vi "autolock.vi"   [LabVIEW 2012]
uses:
  Robot Global Data.vi
  <vilib>/Rock Robotics/WPI/RobotDrive/WPI_RobotDriveGetSetRefNum.vi
types:
  T1 = cluster{"Position":cluster{"X":i32, "Y":i32}, "Distance (ft)":i32, "Center":bool, "Top":bool, "Mid":bool}
  T2 = cluster{"Center Position":cluster{"X":dbl, "Y":dbl}, "Distance (ft)":dbl, "Center":bool, "Top":bool, "Mid":bool}[]
  T3 = typedef "WPI_RobotDriveDevRef.ctl" = cluster{"DevStatus":errorcluster, "Motors[]":T4[], "Square Inputs":bool, "Max Output":dbl, "Isochronous":bool}
  T4 = typedef "WPI_MotorControlDeviceRef.ctl" = cluster{"DeviceStatus":errorcluster, "Type":enum16{"PWM", "CAN"}, "PWM":cluster{"Digital Module":T5, "PWM Channel":T6, "DeadBand":T7}, "CAN":cluster{"Device Number":u8, "Control Mode":T8, "Semaphore":T9, "Max Vout":dbl}, "Invert":bool, "TransformRef":T10, "InvTransformRef":T10}
  T5 = typedef "FPGA_TypedefDigitalModule.ctl" = enum16{"Digital Module 1", "Digital Module 2"}
  T6 = typedef "FPGA_DIOPWMChannel.ctl" = enum8{"PWM 1", "PWM 2", "PWM 3", "PWM 4", "PWM 5", "PWM 6", "PWM 7", "PWM 8", "PWM 9", "PWM 10", "Invalid"}
  T7 = typedef "WPI_PWMDeadband.ctl" = cluster{"Name":string, "maxPositivePwm":i32, "minPositivePwm":i32, "centerPwm":i32, "maxNegativePwm":i32, "minNegativePwm":i32, "angularRange":u16}
  T8 = typedef "WPI_CANJaguar_ControlMode.ctl" = enum8{"Percent VBus", "Current", "Speed", "Position", "Voltage"}
  T9 = typedef "Semaphore RefNum" = refnum<k1>
  T10 = typedef "WPI_PWMTransform_ConPane.ctl" = refnum<vi>
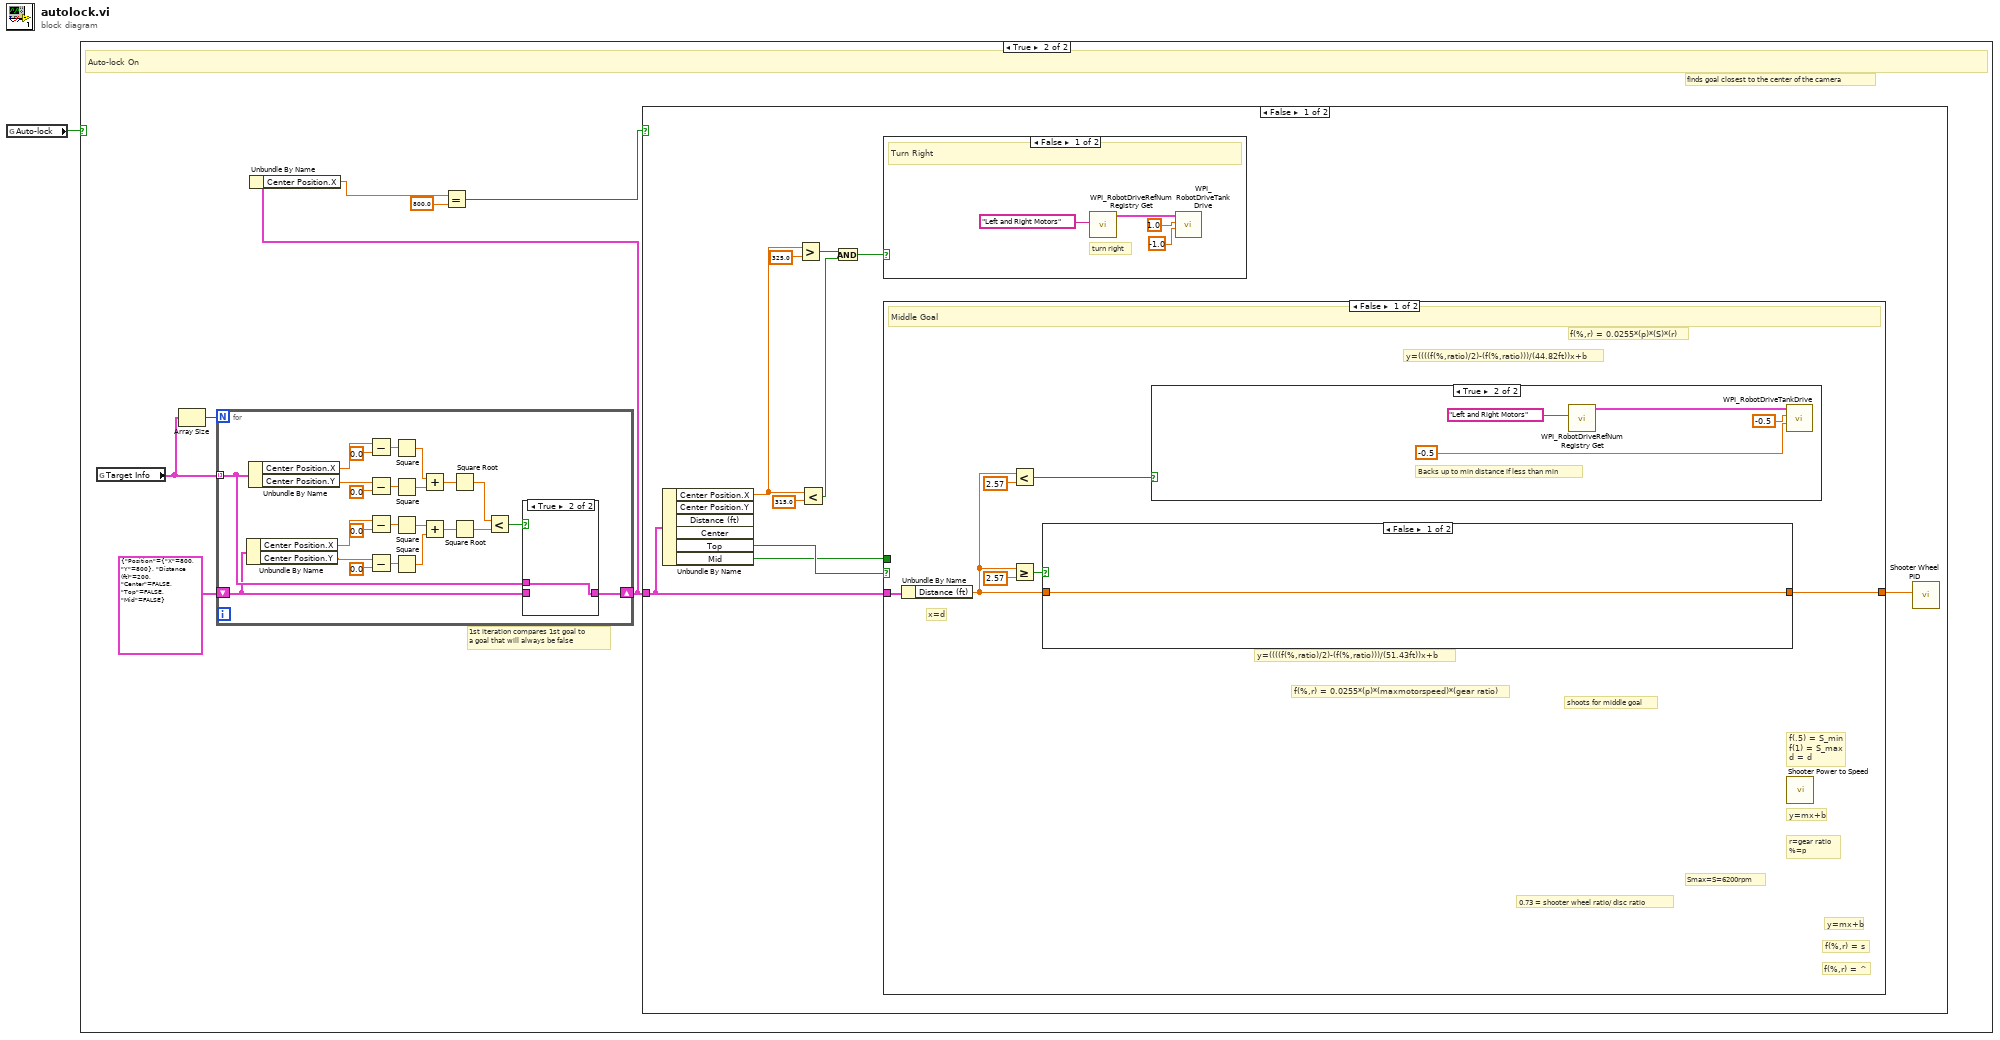
[diagram p0: block diagram]
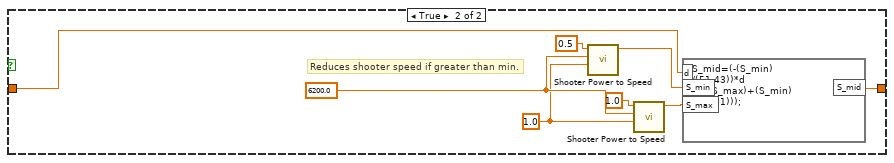
[diagram p4: hidden frame]
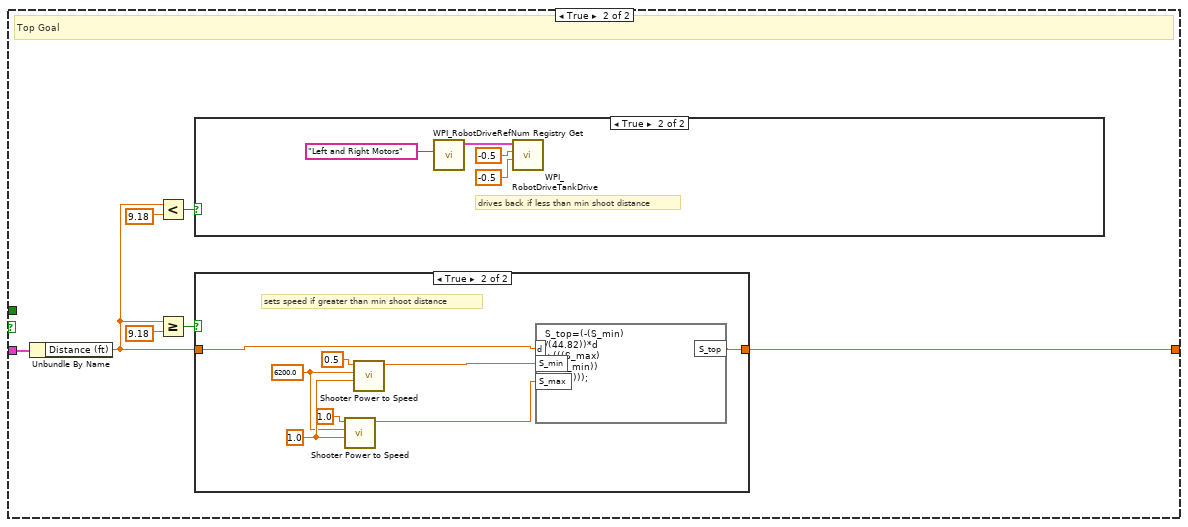
[diagram p5: hidden frame]
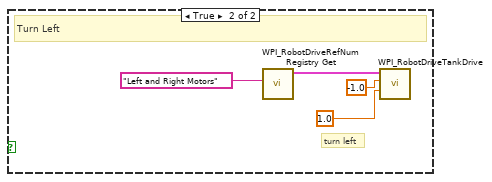
[diagram p8: hidden frame]
diagram:
  n1 = global read "Robot Global Data.vi" "Auto-lock"() -> (w1:bool)
  n2 = case shown="True" w1 {
    frame False {
      # "Auto-lock Off"
    }
    frame True {
      # "1st iteration compares 1st goal to \na goal that will always be false"
      # "finds goal closest to the center of the camera"
      # "Auto-lock On"
      n3 = global read "Robot Global Data.vi" "Target Info"() -> (w7:T2)
      n4 = Array Size(array=w7) -> (size(s)=w8:i32)
      n5 = for {
        N: w8 -> [_]
        tunnel: w7 -> [w82] mode=indexing
        shift-right: [w81] -> w4
        shift-left: T1 {"Position"={"X"=800, "Y"=800}, "Distance (ft)"=200, "Center"=FALSE, "Top"=FALSE, "Mid"=FALSE} -> [w80]
        n6 = Unbundle By Name(w80) -> ("Center Position.X"=w78:dbl, "Center Position.Y"=w75:dbl)
        n7 = Unbundle By Name(w82) -> ("Center Position.X"=w67:dbl, "Center Position.Y"=w71:dbl)
        n8 = Subtract(x=w67, y=0.0) -> (x-y=w68:dbl)
        n9 = Subtract(x=w71, y=0.0) -> (x-y=w70:dbl)
        n10 = Subtract(x=w78, y=0.0) -> (x-y=w76:dbl)
        n11 = Subtract(x=w75, y=0.0) -> (x-y=w73:dbl)
        n12 = Square(x=w68) -> (x^2=w88:dbl)
        n13 = Square(x=w70) -> (x^2=w87:dbl)
        n14 = Square(x=w76) -> (x^2=w86:dbl)
        n15 = Square(x=w73) -> (x^2=w85:dbl)
        n16 = Add(x=w88, y=w87) -> (x+y=w90:dbl)
        n17 = Add(x=w86, y=w85) -> (x+y=w89:dbl)
        n18 = Square Root(x=w90) -> (sqrt(x)=w84:dbl)
        n19 = Square Root(x=w89) -> (sqrt(x)=w83:dbl)
        n20 = Less?(x=w84, y=w83) -> (x < y?=w79:bool)
        n21 = case shown="True" w79 {
          tunnel: w82 -> [_ w92]
          tunnel: [w91 w92] -> w81
          tunnel: w80 -> [w91 _]
          frame False {
          }
          frame True {
          }
        }
      }
      n22 = Unbundle By Name(w4) -> ("Center Position.X"=w3:dbl)
      n23 = Equal?(x=w3, y=800.0) -> (x = y?=w6:bool)
      n24 = case shown="False" w6 {
        tunnel: w4 -> [w13 _]
        frame False {
          n25 = Unbundle By Name(w13) -> ("Center Position.X"=w11:dbl, "Top"=w10:bool, "Mid"=w9:bool)  [unwired: 3 out]
          n26 = Greater?(x=w11, y=325.0) -> (0:w15:bool)
          n27 = Less?(x=w11, y=315.0) -> (x < y?=w16:bool)
          n28 = And(x=w15, y=w16) -> (x .and. y?=w14:bool)
          n29 = case shown="False" w14 {
            frame False {
              # "turn right"
              # "Turn Right"
              n30 = call <vilib>:"WPI_RobotDriveRefNum Registry Get.vi"("refnum name"="Left and Right Motors") -> ("RobotDriveDevRef"=w59:T3)  [unwired: 1 in, 9 out]
              n31 = call <vilib>:"WPI_RobotDriveTankDrive.vi"("Right axis value"=-1.0, "Left axis value"=1.0, "RobotDriveDevRef"=w59) -> ()  [unwired: 6 in, 3 out]
            }
            frame True {
              # "turn left"
              # "Turn Left"
              n32 = call <vilib>:"WPI_RobotDriveRefNum Registry Get.vi"("refnum name"="Left and Right Motors") -> ("RobotDriveDevRef"=w63:T3)  [unwired: 1 in, 9 out]
              n33 = call <vilib>:"WPI_RobotDriveTankDrive.vi"("Right axis value"=1.0, "Left axis value"=-1.0, "RobotDriveDevRef"=w63) -> ()  [unwired: 6 in, 3 out]
            }
          }
          n34 = case shown="False" w10 {
            tunnel: w13 -> [w25 w45]
            tunnel: [w19 w39] -> w12
            tunnel: w9 -> [_ _]
            frame False {
              # "f(.5) = S_min\nf(1) = S_max\nd = d"
              # "y=mx+b"
              # "0.73 = shooter wheel ratio/ disc ratio"
              # "f(%,r) = ^"
              # "x=d"
              # "y=mx+b"
              # "Smax=S=6200rpm"
              # "f(%,r) = 0.0255*(p)*(S)*(r)"
              # "f(%,r) = 0.0255*(p)*(maxmotorspeed)*(gear ratio)"
              # "r=gear ratio\n%=p"
              # "y=((((f(%,ratio)/2)-(f(%,ratio)))/(51.43ft))x+b"
              # "f(%,r) = s"
              # "y=((((f(%,ratio)/2)-(f(%,ratio)))/(44.82ft))x+b"
              # "shoots for middle goal"
              # "Middle Goal"
              n35 = Unbundle By Name(w25) -> ("Distance (ft)"=w20:dbl)
              n36 = Less?(x=w20, y=2.57) -> (x < y?=w22:bool)
              n37 = Greater Or Equal?(x=w20, y=2.57) -> (x >= y?=w21:bool)
              n38 = case shown="False" w21 {
                tunnel: w20 -> [w30 w33]
                tunnel: [w30 w34] -> w19
                frame False {
                }
                frame True {
                  w37 = 6200.0 ("Shooter Maxiimum Speed (rpm)")
                  w36 = 1.0 ("Shooter Wheel/Gear Ratio")
                  # "Reduces shooter speed if greater than min."
                  n39 = call "Shooter Power to Speed.vi"("Shooter Wheel/Gear Ratio"=w36, "Shooter Maxiimum Speed (rpm)"=w37, "Shooter Power (%)"=0.5) -> ("Disc Speed"=w31:dbl)  [unwired: 8 in]
                  n40 = call "Shooter Power to Speed.vi"("Shooter Wheel/Gear Ratio"=w36, "Shooter Maxiimum Speed (rpm)"=w37, "Shooter Power (%)"=1.0) -> ("Disc Speed"=w32:dbl)  [unwired: 8 in]
                  n41 = formula code="S_mid=(-(S_min)\n/(51.43))*d\n+(((S_max)+(S_min)\n/(20.01)));"("d"=w33, "S_min"=w31, "S_max"=w32) -> ("S_mid"=w34:dbl)
                }
              }
              n42 = case shown="True" w22 {
                frame False {
                }
                frame True {
                  # "Backs up to min distance if less than min"
                  n43 = call <vilib>:"WPI_RobotDriveRefNum Registry Get.vi"("refnum name"="Left and Right Motors") -> ("RobotDriveDevRef"=w27:T3)  [unwired: 9 in, 1 out]
                  n44 = call <vilib>:"WPI_RobotDriveTankDrive.vi"("Right axis value"=-0.5, "Left axis value"=-0.5, "RobotDriveDevRef"=w27) -> ()  [unwired: 6 in, 3 out]
                }
              }
              n45 = call "Shooter Power to Speed.vi"() -> ()  [unwired: 11 in, 1 out]
            }
            frame True {
              # "Top Goal"
              n46 = Unbundle By Name(w45) -> ("Distance (ft)"=w40:dbl)
              n47 = Less?(x=w40, y=9.18) -> (x < y?=w41:bool)
              n48 = Greater Or Equal?(x=w40, y=9.18) -> (x >= y?=w44:bool)
              n49 = case shown="True" w41 {
                frame False {
                }
                frame True {
                  # "drives back if less than min shoot distance"
                  n50 = call <vilib>:"WPI_RobotDriveRefNum Registry Get.vi"("refnum name"="Left and Right Motors") -> ("RobotDriveDevRef"=w46:T3)  [unwired: 1 in, 9 out]
                  n51 = call <vilib>:"WPI_RobotDriveTankDrive.vi"("Right axis value"=-0.5, "Left axis value"=-0.5, "RobotDriveDevRef"=w46) -> ()  [unwired: 6 in, 3 out]
                }
              }
              n52 = case shown="True" w44 {
                tunnel: w40 -> [w50 w53]
                tunnel: [w50 w54] -> w39
                frame False {
                }
                frame True {
                  w56 = 6200.0 ("Shooter Maxiimum Speed (rpm)")
                  w57 = 1.0 ("Shooter Wheel/Gear Ratio")
                  # "sets speed if greater than min shoot distance"
                  n53 = call "Shooter Power to Speed.vi"("Shooter Wheel/Gear Ratio"=w57, "Shooter Maxiimum Speed (rpm)"=w56, "Shooter Power (%)"=1.0) -> ("Disc Speed"=w51:dbl)  [unwired: 8 in]
                  n54 = call "Shooter Power to Speed.vi"("Shooter Wheel/Gear Ratio"=w57, "Shooter Maxiimum Speed (rpm)"=w56, "Shooter Power (%)"=0.5) -> ("Disc Speed"=w58:dbl)  [unwired: 8 in]
                  n55 = formula code="S_top=(-(S_min)\n/(44.82))*d\n+(((S_max)\n+((S_min))\n/(4.88)));"("d"=w53, "S_min"=w58, "S_max"=w51) -> ("S_top"=w54:dbl)
                }
              }
            }
          }
          n56 = call "Shooter Wheel PID.vi"("Motor Command (ft/s)"=w12) -> ()  [unwired: 10 in]
        }
        frame True {
        }
      }
    }
  }
